vi "Main.vi"(11 "Module Admin":refnum<class "Delacor_lib_QMH_Module Admin.lvclass">) -> ()   [LabVIEW 2021, in "Control Property Tree.lvlib"]
doc: "This template is based off of the Queued Message Handler design pattern and the Queued Message Handler project template that ships with LabVIEW.\n\nThe main difference is that the queue is private to this module and communication between modules is performed via Broadcast and Request events.\n\nRequest events are wrapped in public API methods and are handled in the Event Handling Loop (EHL) of this VI. Any module can register for Broadcast events sent by this module. The EHL generates messages based on user interface actions.\n\nThe Message Handling Loop (MHL) processes messages generated by the EHL, or by other messages. The messages are string values, so new messages can be added easily to the Message Cases case structure in the MHL. Each message cluster can also provide an optional value for Message Data, which is a variant that can be converted to whatever message-specific data is required.\n_____\nBased on Delacor QMH Project Template 5.0.0.82."
uses:
  Control Property Tree.lvlib
  <vilib>/Delacor/Delacor QMH/Libraries/Module Admin_class/Delacor_lib_QMH_Module Admin.lvclass
  Module Data--cluster.ctl
  Ctrl Properties Map Data.ctl
  Property array.ctl
  Selected Ctrls - List of Controls.ctl
  Selected Ctrls - List of Properties.ctl
  <vilib>/Delacor/Delacor QMH/Libraries/Message Queue_class/Delacor_lib_QMH_Message Queue.lvclass/Delacor_lib_QMH_Message Queue.ctl
  Stop Argument--cluster.ctl
  <vilib>/Delacor/Delacor QMH/Libraries/Module Admin_class/Delacor_lib_QMH_Module Admin.lvclass/Delacor_lib_QMH_Module Admin.ctl
  Load Available PN Argument--cluster.ctl
  Update Property Value Argument--cluster.ctl
  <vilib>/Utility/miscctls.llb/LVPointTypeDef.ctl
  <vilib>/Delacor/Delacor QMH/Libraries/Message Queue_class/Delacor_lib_QMH_Enqueue Message (Single).vi
  <vilib>/Delacor/Delacor QMH/Libraries/Module Admin_class/Delacor_lib_QMH_Get External Launch.vi
  <vilib>/Utility/error.llb/Error Cluster From Error Code.vi
  <vilib>/ErrorRing/Error Ring.xnode
  <vilib>/Delacor/Delacor QMH/Libraries/Message Queue_class/Delacor_lib_QMH_Message Queue.lvclass
  Libraries/Property Panel Launcher/Property Panel Launcher.lvlib
panel:
  in  "Add Control":bool
  in  "Remove Control":bool
  in  "List of Controls":string[](tree)
  in  "List of Properties":string[](tree)
  in  "Simulate MHL Error":bool
  in  "Simulate EHL Error":bool
  out "error out":errorcluster
  out "Status":string
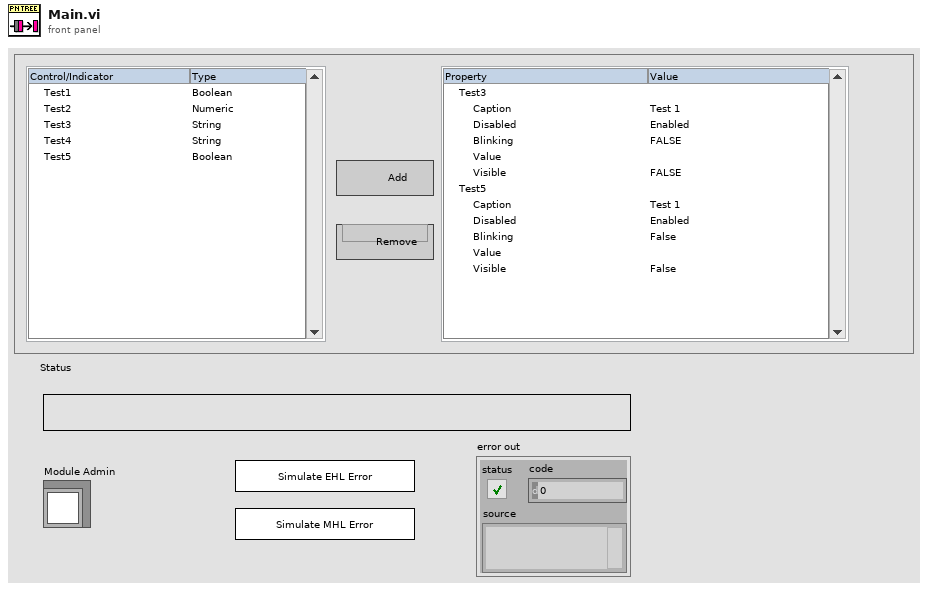
[diagram p1: front panel]
types:
  T1 = typedef "Control Property Tree.lvlib/Request Events--cluster.ctl" = cluster{"Stop Module":refnum<user-event>, "Show Panel":refnum<user-event>, "Hide Panel":refnum<user-event>, "Get Module Execution Status":refnum<user-event>, "Show Diagram":refnum<user-event>, "Load List of Controls":refnum<user-event>, "Load Available PN":refnum<user-event>, "Update Property Value":refnum<user-event>}
  T2 = typedef "Control Property Tree.lvlib/Module Data--cluster.ctl" = cluster{"Status":string, "UI Ctrls":cluster{"Ctrl Names":string[], "Ctrl Types":string[], "Ctrl Tags":string[]}, "Ctrl Properties":map{string, T3}, "Ctrl Properties Template":map{string, T4}, "Temp Data":cluster{"Selected Ctrls - List of Controls":T5, "Selected Ctrls - List of Properties":T6}}
  T3 = typedef "Control Property Tree.lvlib/Ctrl Properties Map Data.ctl" = cluster{"Name":string, "Type":string, "Properties":T4}
  T4 = typedef "Control Property Tree.lvlib/Property array.ctl" = cluster{"Property name":string, "Property tag":string, "Property value (str)":string, "Property value":variant}[]
  T5 = typedef "Control Property Tree.lvlib/Selected Ctrls - List of Controls.ctl" = cluster{"Ctrl Names":string[], "Ctrl Types":string[], "Ctrl Tags":string[]}
  T6 = typedef "Control Property Tree.lvlib/Selected Ctrls - List of Properties.ctl" = cluster{"Ctrl Names":string[], "Ctrl Types":string[], "Ctrl Tags":string[], "Item Indent":i32[], "Property value (str)":string[], "Property value":variant[], "Type of selection":enum16{"No previous selection", "Control selected", "Property selected"}, "Current Selected Property":string}
  T7 = enum32{"invalid lock state", "Not Locked", "Locked (No Password)", "Password-protected"}
  T8 = typedef "Control Property Tree.lvlib/Stop Argument--cluster.ctl" = cluster{"Origin":string, "Exit via Stop Module Req?":bool, "Wait for Module to stop?":bool}
  T9 = typedef "Control Property Tree.lvlib/Load Available PN Argument--cluster.ctl" = cluster{"Boolean":bool}
  T10 = typedef "Control Property Tree.lvlib/Update Property Value Argument--cluster.ctl" = cluster{"Property data":cluster{"Property value":string, "Variant data":variant}}
  T11 = typedef "LVPointTypeDef.ctl" = cluster{"Horizontal":i16, "Vertical":i16}
  T12 = enum32{"Invalid", "Standard", "Closed", "Hidden", "Minimized", "Maximized"}
  T13 = cluster{"Ctrl Names":string[], "Ctrl Types":string[], "Ctrl Tags":string[]}
  T14 = cluster{"Property value":string, "Variant data":variant}
  T15 = cluster{"Left Cell String":string, "Child Text":string[], "Child Tag":string, "Item Indent":i32, "Child Only?":bool, "Glyph Index":i32}[]
  T16 = enum16{"No previous selection", "Control selected", "Property selected"}
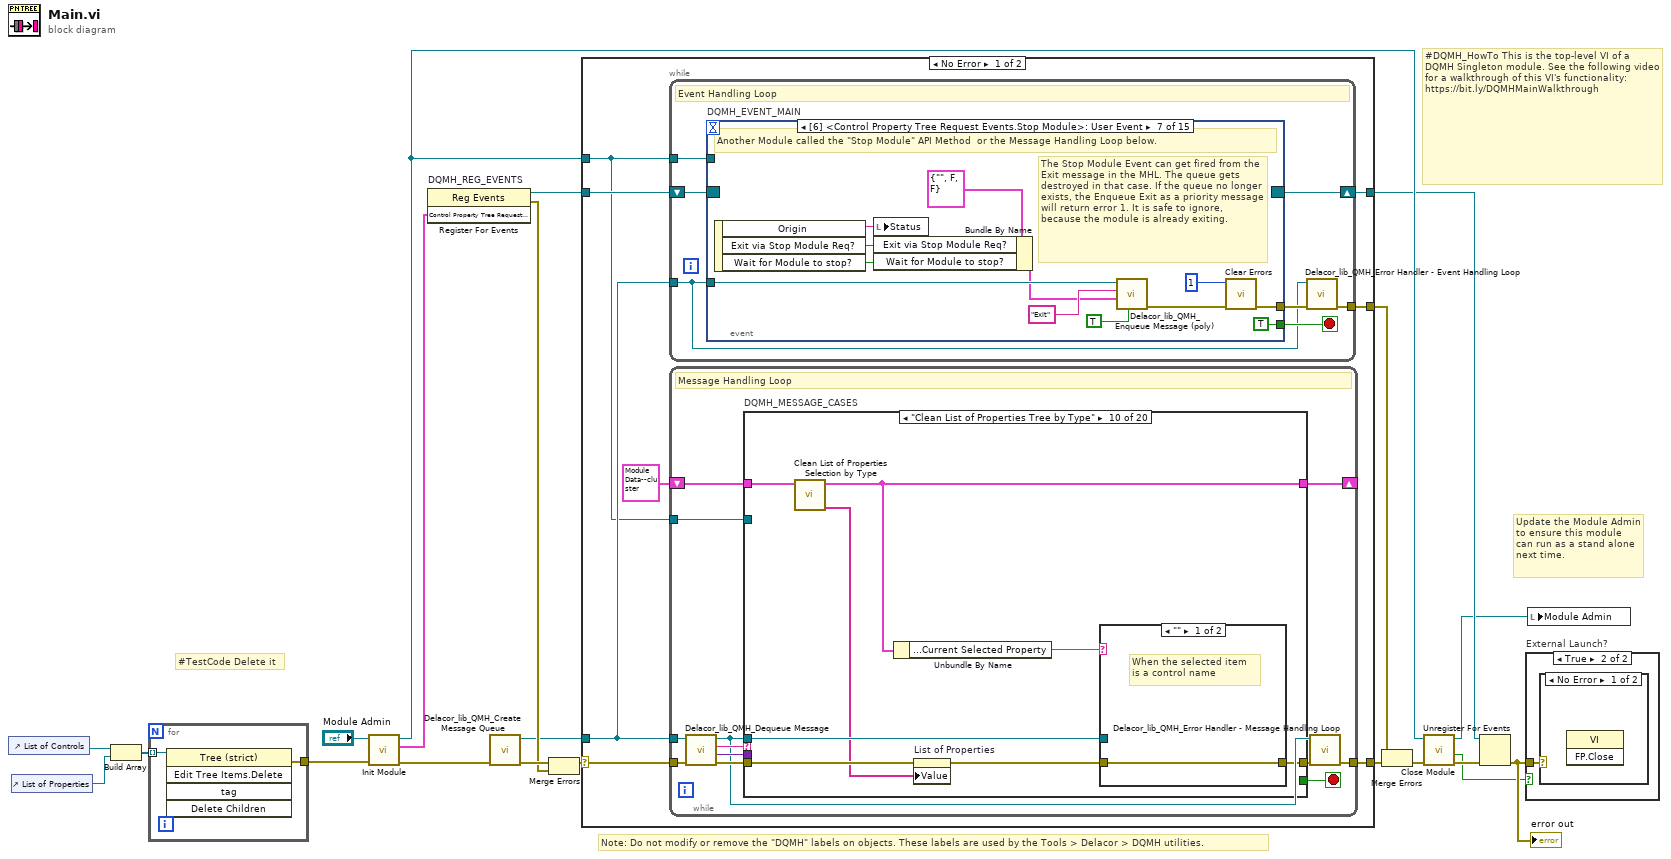
[diagram p0: block diagram]
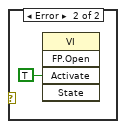
[diagram p3: hidden frame]
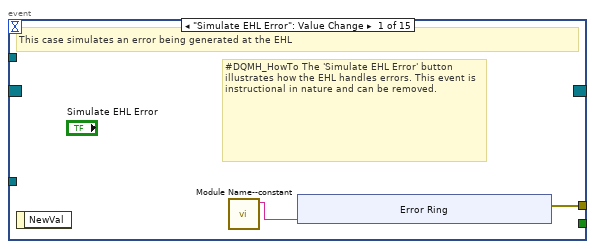
[diagram p4: hidden frame]
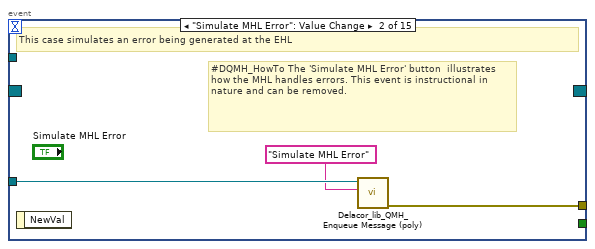
[diagram p5: hidden frame]
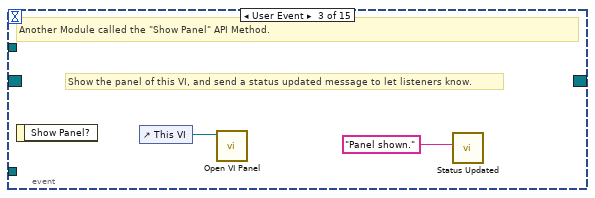
[diagram p6: hidden frame]
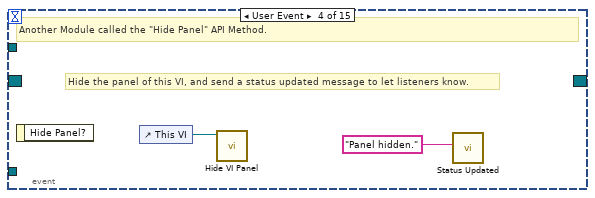
[diagram p7: hidden frame]
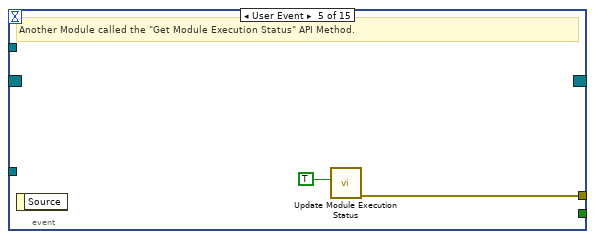
[diagram p8: hidden frame]
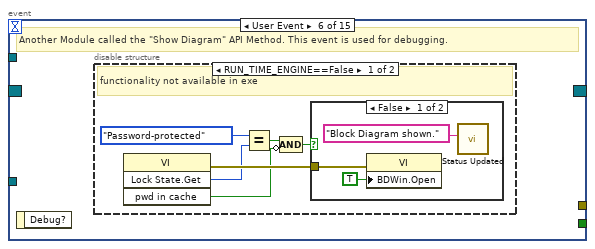
[diagram p9: hidden frame]
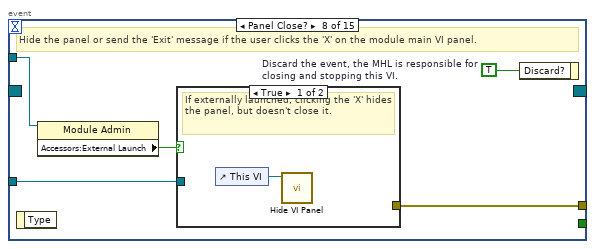
[diagram p12: hidden frame]
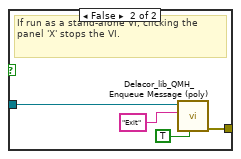
[diagram p13: hidden frame]
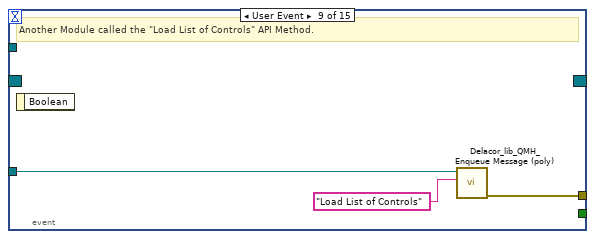
[diagram p14: hidden frame]
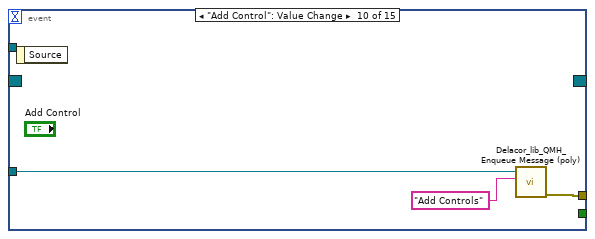
[diagram p15: hidden frame]
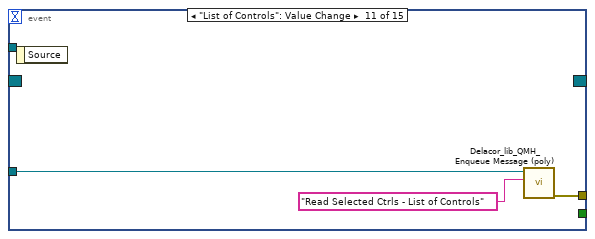
[diagram p16: hidden frame]
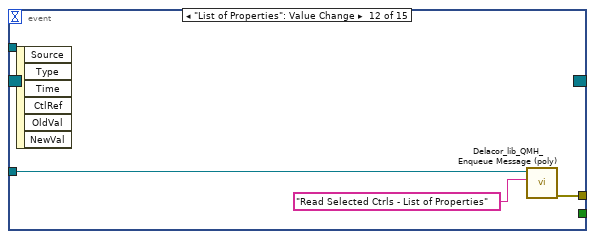
[diagram p17: hidden frame]
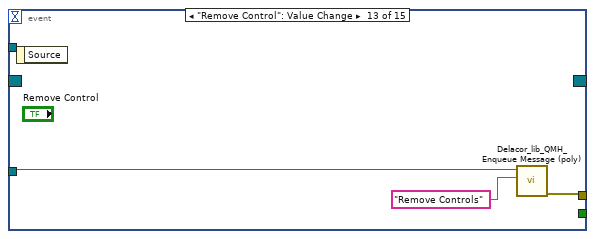
[diagram p18: hidden frame]
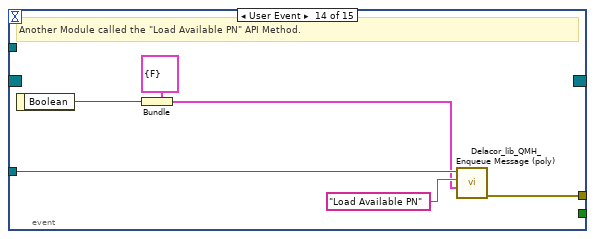
[diagram p19: hidden frame]
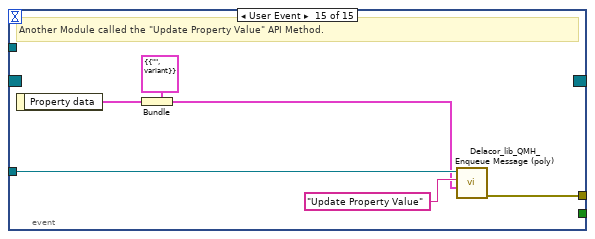
[diagram p20: hidden frame]
diagram:
  # "#TestCode Delete it"
  # "#DQMH_HowTo This is the top-level VI of a DQMH Singleton module. See the following video for a walkthrough of this VI's functionality: https://bit.ly/DQMHMainWalkthrough"
  # "Note: Do not modify or remove the \"DQMH\" labels on objects. These labels are used by the Tools > Delacor > DQMH utilities."
  # "Update the Module Admin to ensure this module can run as a stand alone next time."
  n1 = control-ref of="List of Controls"() -> (w3:refnum<vi>)
  n2 = control-ref of="List of Properties"() -> (w2:refnum<vi>)
  n3 = Build Array(w3, w2) -> (w1:refnum<vi>[])
  n4 = for {
    tunnel: [w23] -> w4
    tunnel: w1 -> [w22] mode=indexing
    n5 = invoke on="Invoke Node" class="Tree (strict)" method="Edit Tree Items.Delete"(reference=w22) -> (error out=w23:errorcluster)  [unwired: 4 in, 4 out]
  }
  n6 = call "Init Module.vi"("error in (no error)"=w4, "Singleton Module Admin in"="Module Admin") -> ("error out"=w20:errorcluster, "Control Property Tree Request Events"=w9:T1, "Singleton Module Admin out"=w12:refnum<class "Delacor_lib_QMH_Module Admin.lvclass">)  [unwired: 7 in]
  n7 = register-events "DQMH_REG_EVENTS"(w9) -> (reference out=w10:refnum<event-registration>, error out=w13:errorcluster)  [unwired: 2 in]
  n8 = call <vilib>:"Delacor_lib_QMH_Create Message Queue.vi"("error in"=w20) -> ("error out"=w15:errorcluster, "Message Queue"=w8:refnum<class "Delacor_lib_QMH_Message Queue.lvclass">)  [unwired: 9 in]
  n9 = Merge Errors(w15, w13) -> (w14:errorcluster)
  n10 = case shown="No Error" w14 {
    selector: w14 -> [w29 w313]
    tunnel: [w31 w312] -> w21
    tunnel: [w28 w318] -> w11
    tunnel: w10 -> [w26 w318]
    tunnel: w8 -> [w25 w311]
    tunnel: [w30 _] -> w18
    tunnel: w12 -> [w24 w314]
    frame No Error {
      n11 = while {
        tunnel: w25 -> [w32]
        shift-right: [w35] -> w28
        shift-left: w26 -> [w36]
        tunnel: [w37] -> w30
        tunnel: w24 -> [w33]
        stop <- w34 stop-if-true
        # "Event Handling Loop"
        n12 = event "DQMH_EVENT_MAIN" shown="[6] <Control Property Tree Request Events.Stop Module>: User Event" {
          selector: w36 -> [_ _ _ _ _ _ _ _ _ _ _ _ _ _ _]
          dyn-events: [_ _ _ _ _ _ _ _ _ _ _ _ _ _ _] -> w35
          timeout: _ -> [_ _ _ _ _ _ _ _ _ _ _ _ _ _ _]
          tunnel: [_ _ _ _ _ _ TRUE ("Discard?") _ _ _ _ _ _ _ _] -> w34
          tunnel: w32 -> [_ w49 _ _ _ _ w73 w80 w90 w92 w94 w98 w100 w108 w114]
          tunnel: [w40 w50 _ _ w56 _ w76 w82 w88 w91 w95 w97 w101 w103 w109] -> w38
          tunnel: w33 -> [_ _ _ _ _ _ _ w79 _ _ _ _ _ _ _]
          event "Simulate EHL Error": Value Change {
            # "#DQMH_HowTo The 'Simulate EHL Error' button  illustrates how the EHL handles errors. This event is instructional in nature and can be removed."
            # "This case simulates an error being generated at the EHL"
            n13 = event-data() -> ()  [unwired: 1 in, 1 out]
            n14 = call "Module Name--constant.vi"() -> ("Module Name"=w39:string)  [unwired: 11 in]
            n15 = xnode "Error Ring"("parameter 0"=w39) -> ("error out"=w40:errorcluster)
          }
          event "Simulate MHL Error": Value Change {
            # "#DQMH_HowTo The 'Simulate MHL Error' button  illustrates how the MHL handles errors. This event is instructional in nature and can be removed."
            # "This case simulates an error being generated at the EHL"
            n16 = event-data() -> ()  [unwired: 1 in, 1 out]
            n17 = call-poly <vilib>:"Delacor_lib_QMH_Enqueue Message (poly).vi"("Message"="Simulate MHL Error", "Message Queue in"=w49) -> ("error out"=w50:errorcluster)  [unwired: 8 in, 1 out]
          }
          event User Event {
            # "Show the panel of this VI, and send a status updated message to let listeners know."
            # "Another Module called the \"Show Panel\" API Method."
            n18 = event-data() -> ()  [unwired: 1 in, 1 out]
            n19 = control-ref of="This VI"() -> (w52:refnum<vi>)
            n20 = call "Open VI Panel.vi"("VI"=w52) -> ()  [unwired: 10 in, 1 out]
            n21 = call "Status Updated.vi"("Status"="Panel shown." ("format string")) -> ()  [unwired: 10 in, 1 out]
          }
          event User Event {
            # "Hide the panel of this VI, and send a status updated message to let listeners know."
            # "Another Module called the \"Hide Panel\" API Method."
            n22 = event-data() -> ()  [unwired: 1 in, 1 out]
            n23 = control-ref of="This VI"() -> (w54:refnum<vi>)
            n24 = call "Hide VI Panel.vi"("VI"=w54) -> ()  [unwired: 10 in, 1 out]
            n25 = call "Status Updated.vi"("Status"="Panel hidden." ("format string")) -> ()  [unwired: 10 in, 1 out]
          }
          event User Event {
            # "Another Module called the \"Get Module Execution Status\" API Method."
            n26 = event-data() -> ()  [unwired: 1 in, 1 out]
            n27 = call "Update Module Execution Status.vi"("Running?"=TRUE) -> ("error out"=w56:errorcluster)  [unwired: 10 in]
          }
          event User Event {
            # "Another Module called the \"Show Diagram\" API Method. This event is used for debugging."
            n28 = event-data() -> ()  [unwired: 1 in, 1 out]
            n29 = disable-structure shown="RUN_TIME_ENGINE==False" {
              frame condition #0 (active) {
                # "functionality not available in exe"
                n30 = invoke class="VI" method="Lock State.Get"() -> (error out=w62:errorcluster, "Get Lock State"=w61:T7, "pwd in cache"=w58:bool)  [unwired: 4 in, 1 out]
                n31 = Equal?(x=T7."Password-protected", y=w61) -> (x = y?=w59:bool)
                n32 = Compound Arithmetic op=AND(w59, invert w58) -> (w57:bool)
                n33 = case shown="False" w57 {
                  tunnel: w62 -> [w65 _]
                  frame False {
                    n34 = property class="VI"(error in=w65, "BDWin.Open"=TRUE ("Block Diagram Window:Open")) -> ()  [unwired: 1 in, 2 out]
                    n35 = call "Status Updated.vi"("Status"="Block Diagram shown." ("format string")) -> ()  [unwired: 10 in, 1 out]
                  }
                  frame True {
                    # "Password-protected VI, and the password is not in the cache. Do not show the diagram."
                  }
                }
              }
              frame condition #1 {
              }
            }
          }
          event User Event {
            # "The Stop Module Event can get fired from the Exit message in the MHL. The queue gets destroyed in that case. If the queue no longer exists, the Enqueue Exit as a priority message will return error 1. It is safe to ignore, because the module is already exiting."
            # "Another Module called the \"Stop Module\" API Method  or the Message Handling Loop below."
            n36 = event-data() -> ("Origin"=w72:string, "Exit via Stop Module Req?"=w68:bool, "Wait for Module to stop?"=w67:bool)  [unwired: 1 in]
            n37 = local write "Status"(w72) -> ()
            n38 = Bundle By Name(cluster=T8 {"Origin"="", "Exit via Stop Module Req?"=FALSE, "Wait for Module to stop?"=FALSE} ("Stop Argument"), "Exit via Stop Module Req?"=w68, "Wait for Module to stop?"=w67) -> (w66:T8)
            n39 = call-poly <vilib>:"Delacor_lib_QMH_Enqueue Message (poly).vi"("Priority Message? (F)"=TRUE, "Message Data"=w66, "Message"="Exit", "Message Queue in"=w73) -> ("error out"=w77:errorcluster)  [unwired: 6 in, 1 out]
            n40 = call <vilib>:"Clear Errors.vi"("error in (no error)"=w77, "specific error code to clear (0: all)"=1) -> ("error out"=w76:errorcluster)  [unwired: 4 in, 1 out]
          }
          event Panel Close? {
            w81 = TRUE  # Discard the event, the MHL is responsible for closing and stopping this VI.
            # "Hide the panel or send the 'Exit' message if the user clicks the 'X' on the module main VI panel."
            n41 = event-data() -> ()  [unwired: 1 in, 1 out]
            n42 = property class="Module Admin"(reference=w79) -> ("Accessors:External Launch"=w78:bool)  [unwired: 1 in, 2 out]
            n43 = case shown="True" w78 {
              tunnel: w80 -> [_ w86]
              tunnel: [_ w87] -> w82
              frame True {
                # "If externally launched, clicking the 'X' hides the panel, but doesn't close it."
                n44 = control-ref of="This VI"() -> (w83:refnum<vi>)
                n45 = call "Hide VI Panel.vi"("VI"=w83) -> ()  [unwired: 10 in, 1 out]
              }
              frame False {
                # "If run as a stand-alone VI, clicking the panel 'X' stops the VI."
                n46 = call-poly <vilib>:"Delacor_lib_QMH_Enqueue Message (poly).vi"("Priority Message? (F)"=TRUE, "Message"="Exit", "Message Queue in"=w86) -> ("error out"=w87:errorcluster)  [unwired: 7 in, 1 out]
              }
            }
            n47 = event-data("Discard?"=w81) -> ()  [unwired: 1 in, 1 out]
          }
          event User Event {
            # "Another Module called the \"Load List of Controls\" API Method."
            n48 = event-data() -> ()  [unwired: 1 in, 1 out]
            n49 = call-poly <vilib>:"Delacor_lib_QMH_Enqueue Message (poly).vi"("Message"="Load List of Controls", "Message Queue in"=w90) -> ("error out"=w88:errorcluster)  [unwired: 8 in, 1 out]
          }
          event "Add Control": Value Change {
            n50 = event-data() -> ()  [unwired: 1 in, 1 out]
            n51 = call-poly <vilib>:"Delacor_lib_QMH_Enqueue Message (poly).vi"("Message"="Add Controls", "Message Queue in"=w92) -> ("error out"=w91:errorcluster)  [unwired: 8 in, 1 out]
          }
          event "List of Controls": Value Change {
            n52 = event-data() -> ()  [unwired: 1 in, 1 out]
            n53 = call-poly <vilib>:"Delacor_lib_QMH_Enqueue Message (poly).vi"("Message"="Read Selected Ctrls - List of Controls", "Message Queue in"=w94) -> ("error out"=w95:errorcluster)  [unwired: 8 in, 1 out]
          }
          event "List of Properties": Value Change {
            n54 = event-data() -> ()  [unwired: 1 in, 6 out]
            n55 = call-poly <vilib>:"Delacor_lib_QMH_Enqueue Message (poly).vi"("Message"="Read Selected Ctrls - List of Properties", "Message Queue in"=w98) -> ("error out"=w97:errorcluster)  [unwired: 8 in, 1 out]
          }
          event "Remove Control": Value Change {
            n56 = event-data() -> ()  [unwired: 1 in, 1 out]
            n57 = call-poly <vilib>:"Delacor_lib_QMH_Enqueue Message (poly).vi"("Message"="Remove Controls", "Message Queue in"=w100) -> ("error out"=w101:errorcluster)  [unwired: 8 in, 1 out]
          }
          event User Event {
            # "Another Module called the \"Load Available PN\" API Method."
            n58 = event-data() -> ("Boolean"=w104:bool)  [unwired: 1 in]
            n59 = Bundle(cluster=T9 {"Boolean"=FALSE} ("Load Available PN Argument"), "Boolean"=w104) -> (w105:T9)
            n60 = call-poly <vilib>:"Delacor_lib_QMH_Enqueue Message (poly).vi"("Message Data"=w105, "Message"="Load Available PN", "Message Queue in"=w108) -> ("error out"=w103:errorcluster)  [unwired: 7 in, 1 out]
          }
          event User Event {
            # "Another Module called the \"Update Property Value\" API Method."
            n61 = event-data() -> ("Property data"=w110:T14)  [unwired: 1 in]
            n62 = Bundle(cluster=T10 {"Property data"={"Property value"="", "Variant data"=variant}} ("Update Property Value Argument"), "Property data"=w110) -> (w111:T10)
            n63 = call-poly <vilib>:"Delacor_lib_QMH_Enqueue Message (poly).vi"("Message Data"=w111, "Message"="Update Property Value", "Message Queue in"=w114) -> ("error out"=w109:errorcluster)  [unwired: 7 in, 1 out]
          }
        }
        n64 = call-dynamic "Delacor_lib_QMH_Error Handler - Event Handling Loop.vi"("error in"=w38, "Message Queue in"=w32) -> ("dup error in"=w37:errorcluster)  [unwired: 8 in, 1 out]
      }
      n65 = while {
        tunnel: w25 -> [w117]
        shift-right: [w121] -> _
        shift-left: T2 {"Status"="", "UI Ctrls"={"Ctrl Names"=[], "Ctrl Types"=[], "Ctrl Tags"=[]}, "Ctrl Properties"={}, "Ctrl Properties Template"={}, "Temp Data"={"Selected Ctrls - List of Controls"={"Ctrl Names"=[], "Ctrl Types"=[], "Ctrl Tags"=[]}, "Selected Ctrls - List of Properties"={"Ctrl Names"=[], "Ctrl Types"=[], "Ctrl Tags"=[], "Item Indent"=[], "Property value (str)"=[], "Property value"=[], "Type of selection"=enum."No previous selection", "Current Selected Property"=""}}} ("Data Cluster") -> [w122]
        tunnel: w29 -> [w125]
        tunnel: [w123] -> w31
        tunnel: w24 -> [w115]
        stop <- w120 stop-if-true
        # "Message Handling Loop"
        n66 = call-dynamic "Delacor_lib_QMH_Dequeue Message.vi"("error in"=w125, "Message Queue in"=w117) -> ("error out"=w124:errorcluster, "Message Data"=w118:variant, "Message"=w119:string, "Message Queue out"=w116:refnum<class "Delacor_lib_QMH_Message Queue.lvclass">)  [unwired: 6 in]
        n67 = case "DQMH_MESSAGE_CASES" shown="\"Clean List of Properties Tree by Type\"" w119 {
          selector: w119 -> [_ _ _ _ _ _ _ _ _ _ _ _ _ _ _ _ _ _ _ w298]
          tunnel: w116 -> [_ _ w150 _ _ w171 _ _ w194 w206 _ w222 _ w239 _ _ _ w268 w290 _]
          tunnel: w124 -> [w144 w148 w152 w158 w165 w170 w178 w189 w201 w209 w219 w223 w233 w248 w251 w253 w258 w275 w296 w300]
          tunnel: [w142 w148 w151 w158 w168 w169 w177 w188 w195 w207 w218 w224 w237 w241 w250 w253 w257 w271 w293 w301] -> w126
          tunnel: w122 -> [w133 w147 w155 w160 w167 w173 w179 w192 w200 w210 w220 w226 w236 w244 w249 w252 w255 w270 w289 w299]
          tunnel: [w132 w147 w153 w159 w167 w173 w174 w191 w202 w204 w220 w225 w236 w242 w249 w252 w255 w270 w289 w299] -> w121
          tunnel: [_ _ _ _ _ _ _ _ _ _ _ _ _ _ _ _ _ _ w288 _] -> w120
          tunnel: w118 -> [_ _ _ _ _ _ _ _ _ _ _ _ _ w247 _ _ _ w269 w287 _]
          tunnel: w115 -> [w134 _ _ _ _ _ _ _ _ _ _ _ _ _ _ _ _ w267 w282 _]
          frame "Initialize" {
            w127 = "Initial Message" ("Initial Message")
            # "#CodeNeeded - Initialize the appearance of the front panel."
            # "#CodeNeeded - Initialize your state data here."
            # "Initialize - Any operation that needs to be done before the module can receive messages. Synchronize Caller Events.vi will inform Start Module.vi that the module has launched and is ready to receive messages. Module Did Init.vi will broadcast that the module initialized."
            n68 = call "Synchronize Caller Events.vi"("error in (no error)"=w144, "Singleton Module Admin in"=w134) -> ("error out"=w143:errorcluster, "Singleton Module Admin out"=w129:refnum<class "Delacor_lib_QMH_Module Admin.lvclass">)  [unwired: 8 in]
            n69 = property class="Module Admin"(reference=w129) -> ("Accessors:External Launch"=w138:bool)  [unwired: 1 in, 2 out]
            n70 = invoke class="VI" method="Default Vals.Reinit All"() -> ()  [unwired: 3 in, 3 out]
            n71 = Select(t=T12."Hidden" ("State"), s=w138, f=T12."Standard" ("State")) -> (s? t:f=w135:T12)
            n72 = call "Module Name--constant.vi"() -> ("Module Name"=w141:string)  [unwired: 11 in]
            n73 = property class="VI"("Front Panel.Title"=w141) -> (reference out=w140:refnum<vi>, error out=w146:errorcluster)  [unwired: 2 in]
            n74 = call "Module Name--constant.vi"() -> ("Module Name"=w130:string)  [unwired: 11 in]
            n75 = invoke class="VI" method="FP.Open"(reference=w140, error in=w146, "State"=w135) -> (reference out=w139:refnum<vi>, error out=w145:errorcluster)  [unwired: 2 in, 3 out]
            n76 = Bundle By Name(cluster=w133, "Status"=w127) -> (w132:T2)
            n77 = call "Module Did Init.vi"("error in (no error)"=w143, "Initialized?"=TRUE, "Origin"=w130) -> ("error out"=w142:errorcluster)  [unwired: 8 in]
            n78 = invoke class="VI" method="FP.Center"(reference=w139, error in=w145) -> ()  [unwired: 1 in, 3 out]
            n79 = property on="Pane" class="Pane"("Origin"=T11 {"Horizontal"=0, "Vertical"=0}) -> ()  [unwired: 2 in, 2 out]
            "Status" <- w127
          }
          frame "--- Module Specific ---" {
            # "Separator -- The following cases handle messages specific to this Module."
          }
          frame "Load List of Controls" {
            # "Loads the controls (names and types) into the List of Controls tree."
            n80 = Bundle By Name(cluster=w155, "UI Ctrls"=T13 {"Ctrl Names"=["Test1", "Test2", "Test3", "Test4", "Test5"], "Ctrl Types"=["Boolean", "Numeric", "String", "String", "Boolean"], "Ctrl Tags"=["TagTest1", "TagTest2", "TagTest3", "TagTest4", "TagTest5"]}) -> (w153:T2)
            n81 = call-poly <vilib>:"Delacor_lib_QMH_Enqueue Message (poly).vi"("error in"=w152, "Message"="Update List of Controls", "Message Queue in"=w150) -> ("error out"=w151:errorcluster)  [unwired: 7 in, 1 out]
          }
          frame "Load Available PN" {
            w156 = T4 [{"Property name"="Caption", "Property tag"="Caption", "Property value (str)"="Test 1", "Property value"=variant}, {"Property name"="Disabled", "Property tag"="Disabled", "Property value (str)"="Enabled", "Property value"=variant}, {"Property name"="Blinking", "Property tag"="Blinking", "Property value (str)"="False", "Property value"=variant}, {"Property name"="Value", "Property tag"="Value", "Property value (str)"="", "Property value"=variant}, {"Property name"="Visible", "Property tag"="Visible", "Property value (str)"="False", "Property value"=variant}] ("Properties")
            # "Test code"
            n82 = node("Boolean" ("key"), w156, "Numeric" ("key"), w156, "String" ("key"), w156) -> (w157:map{string, T4})
            n83 = Bundle By Name(cluster=w160, "Ctrl Properties Template"=w157) -> (w159:T2)
          }
          frame "Update List of Controls" {
            n84 = call "Update List of Controls Tree.vi"("error in (no error)"=w165, "Data Cluster"=w167) -> ("error out"=w164:errorcluster, "Items"=w166:T15)  [unwired: 8 in]
            n85 = invoke on="List of Controls" class="Tree (strict)" method="Edit Tree Items.Add Multiple Items to End"(error in=w164, "Items"=w166) -> (error out=w168:errorcluster)  [unwired: 2 in, 3 out]
          }
          frame "Add Controls" {
            n86 = call-poly <vilib>:"Delacor_lib_QMH_Enqueue Message (poly).vi"("error in"=w170, "Message"="Add to Ctrl Properties", "Message Queue in"=w171) -> ("error out"=w169:errorcluster)  [unwired: 7 in, 1 out]
          }
          frame "Remove Controls" {
            n87 = call "Remove Controls from List of Properties.vi"("Data Cluster in"=w179) -> ("Type of selection"=w175:T16, "Ctrl Tags"=w176:string[], "Data Cluster out"=w174:T2)  [unwired: 8 in]
            n88 = case shown="\"Control selected\"" w175 {
              tunnel: w178 -> [w180 w182]
              tunnel: w176 -> [_ w183]
              tunnel: [w180 w181] -> w177
              frame "No previous selection", Default {
              }
              frame "Control selected" {
                n89 = for {
                  tunnel: w183 -> [w186] mode=indexing
                  shift-right: [w184] -> w181
                  shift-left: w182 -> [w185]
                  n90 = invoke on="List of Properties" class="Tree (strict)" method="Edit Tree Items.Delete"(error in=w185, "tag"=w186, "Delete Children"=TRUE ("Delete Children?")) -> (error out=w184:errorcluster)  [unwired: 2 in, 4 out]
                }
              }
            }
          }
          frame "Read Selected Ctrls - List of Controls" {
            n91 = call "Get Selected Controls.vi"("error in (no error)"=w189, "List of Properties"="List of Controls", "Data in"=w192) -> ("error out"=w188:errorcluster, "Selected Ctrls"=w190:T13)  [unwired: 7 in]
            n92 = Bundle By Name(cluster=w192, "Temp Data.Selected Ctrls - List of Controls"=w190) -> (w191:T2)
          }
          frame "Read Selected Ctrls - List of Properties" {
            n93 = call "Get Selected Controls - List of properties.vi"("error in (no error)"=w201, "List of Properties"="List of Properties", "Data in"=w200) -> ("error out"=w196:errorcluster, "Selected Ctrls - List of Properties"=w198:T6)  [unwired: 7 in]
            n94 = Bundle By Name(cluster=w200, "Temp Data.Selected Ctrls - List of Properties"=w198) -> (w202:T2)
            n95 = call-poly <vilib>:"Delacor_lib_QMH_Enqueue Message (poly).vi"("error in"=w196, "Message"="Clean List of Properties Tree by Type", "Message Queue in"=w194) -> ("error out"=w195:errorcluster)  [unwired: 7 in, 1 out]
          }
          frame "Clean List of Properties Tree by Type" {
            n96 = call "Clean List of Properties Selection by Type.vi"("Data Cluster in"=w210) -> ("List of Tags"=w205:string[], "output cluster"=w204:T2)  [unwired: 9 in]
            n97 = Unbundle By Name(w204) -> ("Temp Data.Selected Ctrls - List of Properties.Current Selected Property"=w203:string)
            n98 = property on="List of Properties" class="Tree (strict)"(error in=w209, "Value"=w205) -> (error out=w208:errorcluster)  [unwired: 1 in, 1 out]
            n99 = case shown="\"\"" w203 {
              tunnel: w208 -> [w211 w214]
              tunnel: [w211 w213] -> w207
              tunnel: w206 -> [_ w212]
              frame "" {
                # "When the selected item \nis a control name"
              }
              frame Default {
                # "When the selected item\nis a property name"
                n100 = call-poly <vilib>:"Delacor_lib_QMH_Enqueue Message (poly).vi"("error in"=w214, "Message"="Load Property Subpanel", "Message Queue in"=w212) -> ("error out"=w213:errorcluster)  [unwired: 7 in, 1 out]
              }
            }
          }
          frame "Load Property Subpanel" {
            n101 = Unbundle By Name(w220) -> ("Temp Data.Selected Ctrls - List of Properties.Current Selected Property"=w217:string, "Temp Data.Selected Ctrls - List of Properties.Property value"=w216:variant[])
            n102 = call "Load Panel.vi"("error in (no error)"=w219, "Property values"=w216, "Current Selected Property"=w217) -> ("error out"=w218:errorcluster)  [unwired: 8 in]
          }
          frame "Add to Ctrl Properties" {
            n103 = call "Add Selected Ctrl Properties.vi"("Data Cluster In"=w226) -> ("New data?"=w221:bool, "Data Cluster out"=w225:T2)  [unwired: 9 in]
            n104 = case shown="False" w221 {
              tunnel: [w227 w230] -> w224
              tunnel: w223 -> [w227 w229]
              tunnel: w222 -> [_ w228]
              frame False {
              }
              frame True {
                n105 = call-poly <vilib>:"Delacor_lib_QMH_Enqueue Message (poly).vi"("error in"=w229, "Message"="Update List of Properties", "Message Queue in"=w228) -> ("error out"=w230:errorcluster)  [unwired: 7 in, 1 out]
              }
            }
          }
          frame "Update List of Properties" {
            n106 = invoke on="List of Properties" class="Tree (strict)" method="Edit Tree Items.Delete"(error in=w233) -> (error out=w232:errorcluster)  [unwired: 4 in, 4 out]
            n107 = call "Convert to Tree Data.vi"("error in (no error)"=w232, "Data Cluster"=w236) -> ("error out"=w234:errorcluster, "Items out"=w235:T15)  [unwired: 8 in]
            n108 = invoke on="List of Properties" class="Tree (strict)" method="Edit Tree Items.Add Multiple Items to End"(error in=w234, "Items"=w235) -> (error out=w237:errorcluster)  [unwired: 2 in, 3 out]
          }
          frame "Update Property Value" {
            # "Updates the Selected Property value with the data coming from the Property Panel"
            n109 = Variant To Data(error in=w248, type=T10 {"Property data"={"Property value"="", "Variant data"=variant}} ("Update Property Value Argument"), Variant=w247) -> (data=w245:T10, error out=w240:errorcluster)
            n110 = Unbundle By Name(w245) -> ("Property data"=w243:T14)
            n111 = call "Update Property Map Value.vi"("Property data in"=w243, "Data Cluster in"=w244) -> ("Data Cluster out"=w242:T2)  [unwired: 9 in]
            n112 = call-poly <vilib>:"Delacor_lib_QMH_Enqueue Message (poly).vi"("error in"=w240, "Message"="Update List of Properties", "Message Queue in"=w239) -> ("error out"=w241:errorcluster)  [unwired: 7 in, 1 out]
          }
          frame "---Copy This Frame---" {
            # "Duplicate this frame when creating new messages.  Change this comment in the duplicated frame to describe this message."
            n113 = Merge Errors(w251) -> (w250:errorcluster)
          }
          frame "--- Exit and Error Handling---" {
            # "Separator - The following cases handle errors and exit messages."
          }
          frame "Simulate MHL Error" {
            # "#DQMH_HowTo The 'Simulate MHL Error' button  illustrates how the MHL handles errors. This event is instructional in nature and can be removed."
            # "Simulate an error occurring at the MHL"
            n114 = call "Module Name--constant.vi"() -> ("Module Name"=w254:string)  [unwired: 11 in]
            n115 = xnode "Error Ring"("parameter 0"=w254) -> ("error out"=w256:errorcluster)
            n116 = Merge Errors(w258, w256) -> (w257:errorcluster)
          }
          frame "Error" {
            # "#CodeRecommended - If you ever change the name of this \"Error\" message, you'll need to update the name in the Check Loop Error.vi as well."
            # "#CodeRecommended - If the module is running in standalone mode (External Launch = FALSE), this code will pop up an error dialog and call the 'Exit' message if an error occurs. Add more fine-grained error handling here."
            # "Error - Check the error message data and respond accordingly. This message is sent by the \"Error Handler\" VIs at the end of each loop in this application."
            n117 = property class="Module Admin"(reference=w267) -> ("Accessors:External Launch"=w266:bool)  [unwired: 1 in, 2 out]
            n118 = Variant To Data(error in=w275, type=errorcluster {"status"=FALSE, "code"=0, "source"=""} ("error constant"), Variant=w269) -> (data=w276:errorcluster, error out=w273:errorcluster)
            n119 = call "Error Reported.vi"("Error"=w276) -> ()  [unwired: 10 in, 1 out]
            n120 = case shown="False" w266 {
              tunnel: [w281 _] -> w272
              tunnel: w268 -> [w279 _]
              tunnel: w276 -> [w280 _]
              frame False {
                # "If the module is running standalone, then pop up an error dialog and call the \"Exit\" message."
                n121 = call <vilib>:"Simple Error Handler.vi"("error in (no error)"=w280) -> ()  [unwired: 4 in, 5 out]
                n122 = call-poly <vilib>:"Delacor_lib_QMH_Enqueue Message (poly).vi"("Priority Message? (F)"=TRUE, "Message"="Exit", "Message Queue in"=w279) -> ("error out"=w281:errorcluster)  [unwired: 7 in, 1 out]
              }
              frame True {
                # "If the module was launched externally, calling the Error Reported broadcast VI is the only action performed by the \"Error\" message. The module's caller can then process the error appropriately."
              }
            }
            n123 = Merge Errors(w273, w272) -> (w271:errorcluster)
            n124 = local write "error out"(w271) -> ()
          }
          frame "Exit" {
            w286 = 91  # 91: not all Exit messages will have an argument
            w288 = TRUE  # Stop the VI
            # "Release the message queue reference"
            # "#CodeNeeded - Add any required cleanup code here"
            # "Exit - Exit the application."
            n125 = Variant To Data(error in=w296, type=T8 {"Origin"="", "Exit via Stop Module Req?"=FALSE, "Wait for Module to stop?"=FALSE} ("Stop Argument"), Variant=w287) -> (data=w284:T8, error out=w292:errorcluster)
            n126 = call <vilib>:"Clear Errors.vi"("error in (no error)"=w292, "specific error code to clear (0: all)"=w286) -> ("error out"=w295:errorcluster)  [unwired: 4 in, 1 out]
            n127 = control-ref of="This VI"() -> (w283:refnum<vi>)
            n128 = call-dynamic "Delacor_lib_QMH_Release Message Queue.vi"("error in"=w295, "Message Queue"=w290) -> ("error out"=w294:errorcluster)  [unwired: 9 in]
            n129 = call "Handle Exit.vi"("Stop Argument"=w284, "Admin in"=w282, "VI reference"=w283) -> ("error out"=w291:errorcluster)  [unwired: 7 in, 1 out]
            n130 = Merge Errors(w294, w291) -> (w293:errorcluster)
          }
          frame Default {
            # "'Default' case only runs if there is a message that isn't defined in any of the other cases.  Output a programming error."
            n131 = call "Module Name--constant.vi"() -> ("Module Name"=w297:string)  [unwired: 11 in]
            n132 = xnode "Error Ring"("parameter 0"=w298, "parameter 1"=w297) -> ("error out"=w302:errorcluster)
            n133 = Merge Errors(w300, w302) -> (w301:errorcluster)
          }
        }
        n134 = call-dynamic "Delacor_lib_QMH_Error Handler - Message Handling Loop.vi"("error in"=w126, "Message Queue in"=w116) -> ("dup error in"=w123:errorcluster)  [unwired: 8 in, 1 out]
      }
    }
    frame Error {
      # "Synchronize Caller Events.vi will inform Start Module.vi that the module has launched and will let the code calling Start Module.vi register for broadcasts and would permit the caller receive the broadcast that an error occurred at launch time."
      n135 = call-dynamic "Delacor_lib_QMH_Release Message Queue.vi"("error in"=w313, "Message Queue"=w311) -> ("error out"=w312:errorcluster)  [unwired: 9 in]
      n136 = call "Synchronize Caller Events.vi"("Singleton Module Admin in"=w314) -> ("error out"=w319:errorcluster)  [unwired: 9 in, 1 out]
      n137 = call "Module Name--constant.vi"() -> ("Module Name"=w317:string)  [unwired: 11 in]
      n138 = Format Into String(format string="An error occurred during initialization. %s is no longer running.", w317) -> (resulting string=w315:string)  [unwired: 2 in, 1 out]
      n139 = Merge Errors(w312, w319) -> (w320:errorcluster)
      n140 = call "Error Reported.vi"("Additional Information"=w315, "Error"=w320) -> ()  [unwired: 9 in, 1 out]
    }
  }
  n141 = Merge Errors(w18, w21) -> (w17:errorcluster)
  n142 = call "Close Module.vi"("error in (no error)"=w17, "Module Admin in"=w12) -> ("error out"=w19:errorcluster, "External Launch"=w5:bool, "Module Admin out"=w6:refnum<class "Delacor_lib_QMH_Module Admin.lvclass">)  [unwired: 7 in]
  n143 = Unregister For Events(event registration refnum=w11, error in=w19) -> (error out=w16:errorcluster)
  "error out" <- w16
  n144 = case "External Launch?" shown="True" w5 {
    tunnel: w16 -> [_ w321]
    frame False {
    }
    frame True {
      n145 = case shown="No Error" w321 {
        frame No Error {
          n146 = invoke class="VI" method="FP.Close"() -> ()  [unwired: 3 in, 3 out]
        }
        frame Error {
          n147 = invoke class="VI" method="FP.Open"("Activate"=TRUE ("Activate?")) -> ()  [unwired: 4 in, 5 out]
        }
      }
    }
  }
  n148 = local write "Module Admin"(w6) -> ()
